vi "Format Path.vi"(11 "Input path":path) -> (3 "Output path":path)   [LabVIEW 2012, in "AcquisitionCoreObjects.lvlib" / "AcquistionObject.lvclass"]
uses:
  AcquistionObject.lvclass
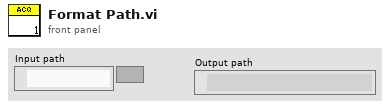
[diagram p1: front panel]
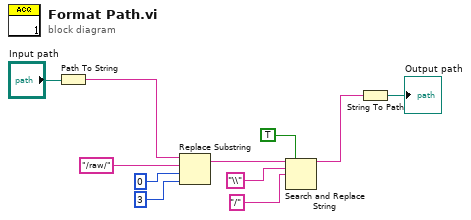
[diagram p0: block diagram]
diagram:
  n1 = Path To String(path="Input path") -> (string=w4:string)
  n2 = Replace Substring(2:3 ("length (len. of substring)"), 3:0 ("offset (0)"), 4:"/raw/" ("substring (\"\")"), 5:w4) -> (1:w8:string)  [unwired: 1 out]
  n3 = Search and Replace String(replace all?=TRUE ("replace all? (F)"), input string=w8, search string="\\", replace string="/" ("replace string (\"\")")) -> (result string=w3:string)  [unwired: 4 in, 3 out]
  n4 = String To Path(string=w3) -> (path=→"Output path":path)
